vi "Save Config User Event (by ref).vi"(10 "Graph Settings":T1, 11 "Register (F)":bool) -> (3 "Save Config Event Ref":refnum<user-event>)   [LabVIEW 2019]
uses:
  Type Defs and Controls/Graph Settings Type Def.ctl
  Type Defs and Controls/Save Config Event Type Def.ctl
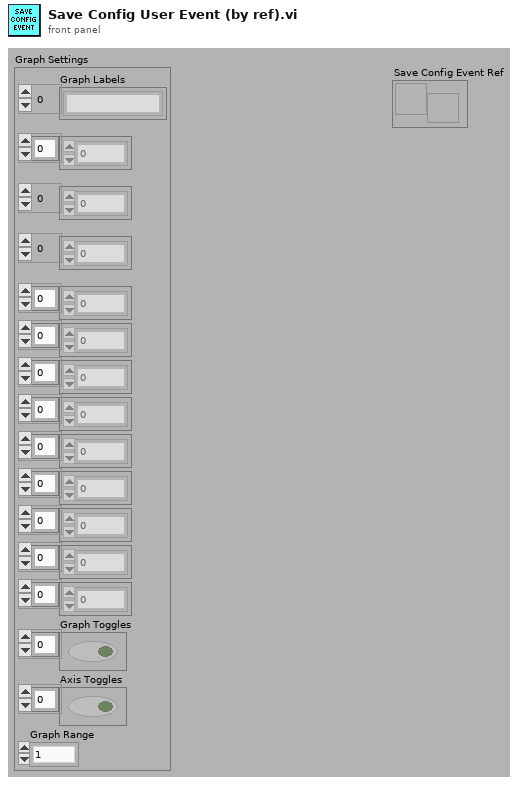
[diagram p1: front panel]
types:
  T1 = typedef "Graph Settings Type Def.ctl" = cluster{"Graph Labels":string[], u8[], i16[], u32[], u8[], u8[], u8[], u32[], u8[], u8[], u8[], dbl[], dbl[], "Graph Toggles":bool[], "Axis Toggles":bool[], "Graph Range":enum16{"1", "2", "3", "4", "5", "10", "15", "30", "60"}}
  T2 = typedef "Save Config Event Type Def.ctl" = cluster{"Graph Settings":T1}
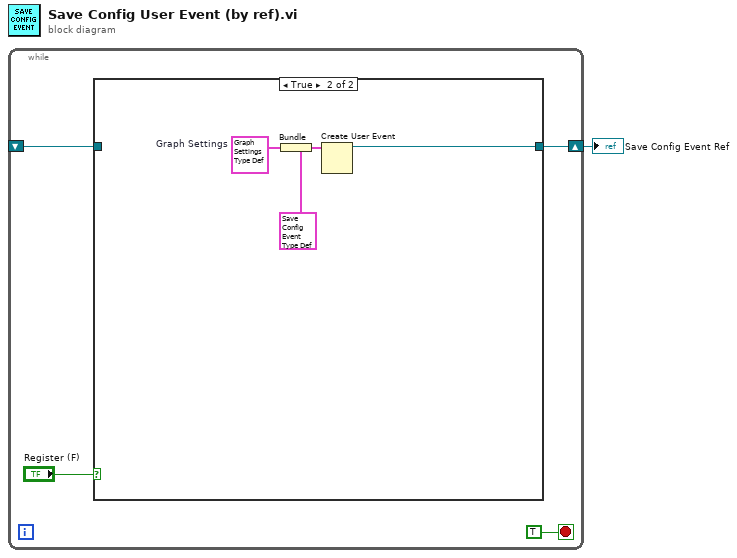
[diagram p0: block diagram]
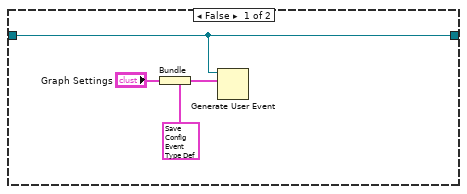
[diagram p2: hidden frame]
diagram:
  n1 = while {
    shift-right: [w3] -> w1
    shift-left: _ -> [w2]
    stop <- TRUE stop-if-true
    n2 = case shown="True" "Register (F)" {
      tunnel: [w9 w13] -> w3
      tunnel: w2 -> [w9 _]
      frame False {
        n3 = Bundle(cluster=T2 {"Graph Settings"={"Graph Labels"=[], [], [], [], [], [], [], [], [], [], [], [], [], "Graph Toggles"=[], "Axis Toggles"=[], "Graph Range"=enum."1"}} ("Save Config Event Type Def"), "Graph Settings"="Graph Settings") -> (w8:T2)
        n4 = Generate User Event(user event=w9, event data cluster=w8) -> ()  [unwired: 2 in, 2 out]
      }
      frame True {
        w12 = T1 {"Graph Labels"=[], [], [], [], [], [], [], [], [], [], [], [], [], "Graph Toggles"=[], "Axis Toggles"=[], "Graph Range"=enum."1"}  # Graph Settings
        n5 = Bundle(cluster=T2 {"Graph Settings"={"Graph Labels"=[], [], [], [], [], [], [], [], [], [], [], [], [], "Graph Toggles"=[], "Axis Toggles"=[], "Graph Range"=enum."1"}} ("Save Config Event Type Def"), "Graph Settings"=w12) -> (w10:T2)
        n6 = Create User Event(user event datatype=w10) -> (user event=w13:refnum<user-event>)  [unwired: 1 in, 1 out]
      }
    }
  }
  "Save Config Event Ref" <- w1
